vi "chart axis set log base.vi"(8 "error in (no error)":errorcluster, 10 "log_base":u16, 11 "axis":u32) -> (0 "error out":errorcluster)   [LabVIEW 2015, in "xlsxwriter.lvlib"]
doc: "void chart_axis_set_log_base(lxw_chart_axis axis, uint16_t log_base);"
uses:
  xlsxwriter.lvlib
  xlsxwriter.dll
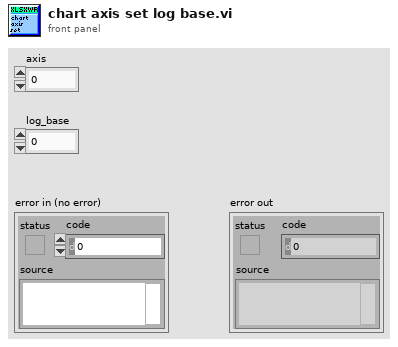
[diagram p1: front panel]
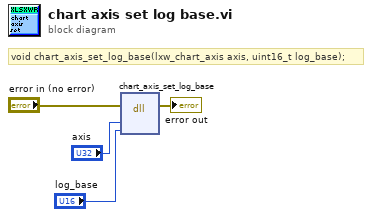
[diagram p0: block diagram]
diagram:
  # "void chart_axis_set_log_base(lxw_chart_axis axis, uint16_t log_base);"
  n1 = dll-call lib="C:/Users/WDAGUtilityAccount/Desktop/lv_vis_added_cell/xlsxwriter.*" fn="chart_axis_set_log_base"(error in="error in (no error)", "axis"="axis", "log_base"="log_base") -> (error out=→"error out":errorcluster)  [unwired: 5 in, 1 out]
